vi "Get Time.vi"(11 "Class 2.lvclass":refnum<class "Class 2.lvclass">) -> (2 "change":bool, 3 "Class 2.lvclass 2":refnum<class "Class 2.lvclass">)   [LabVIEW 2019, in "Class 2.lvclass"]
uses:
  Class 2.lvclass
  Class 2.lvclass/Class 2.ctl
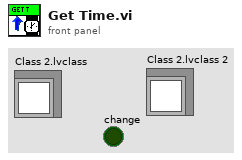
[diagram p1: front panel]
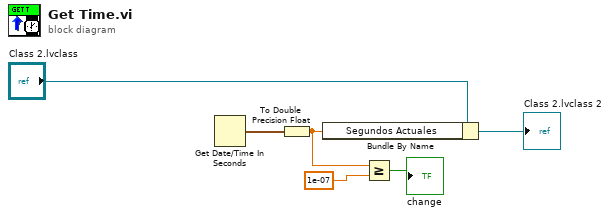
[diagram p0: block diagram]
diagram:
  n1 = Get Date/Time In Seconds() -> (seconds since 1Jan1904=w6:timestamp)
  n2 = To Double Precision Float(number=w6) -> (double precision float=w3:dbl)
  n3 = Bundle By Name(cluster="Class 2.lvclass", "Segundos Actuales"=w3) -> (→"Class 2.lvclass 2":refnum<class "Class 2.lvclass">)
  n4 = Greater Or Equal?(x=w3, y=1e-07) -> (x >= y?=→"change":bool)
